vi "Choreo_ChoreoDifferential_LoadTrajectoryString.vi"(11 "trajectoryJsonString":string) -> (0 "Error":bool, 3 "ChoreoTrajectoryDifferential":T1)   [LabVIEW 2019, in "ChoreoLib.lvlib"]
doc: "Parse a Differential choreo trajectory from a JSON formatted string. \n\nInputs: \n - trajectoryJsonString - string- The string containing the choreo trajectory. Note that files may have a .TRAJ extension. These are actually internally formatted as JSON files.\n\nOutputs:\n - ChoreoTrajectorySwerve - cluster - Trajectory read from JSON file.\n - Error - boolean - TRUE if an error occured."
uses:
  ChoreoLib.lvlib
  TypeDef/ChoreoEventMarker.ctl
  TypeDef/ChoreoTrajectoryDifferential.ctl
  TypeDef/ChoreoDifferentialSample.ctl
panel:
  out "nameErr":bool
  out "EventsEmpty":bool
  out "EventMarkers":T3[](array[typedef])
  out "splitsErr":bool
  out "version":i32
  out "sampleType":string
  out "VersionErr":bool
  out "SampleTypeErr":bool
  in  "?":T4(array[cluster])
  out "sampleError":bool
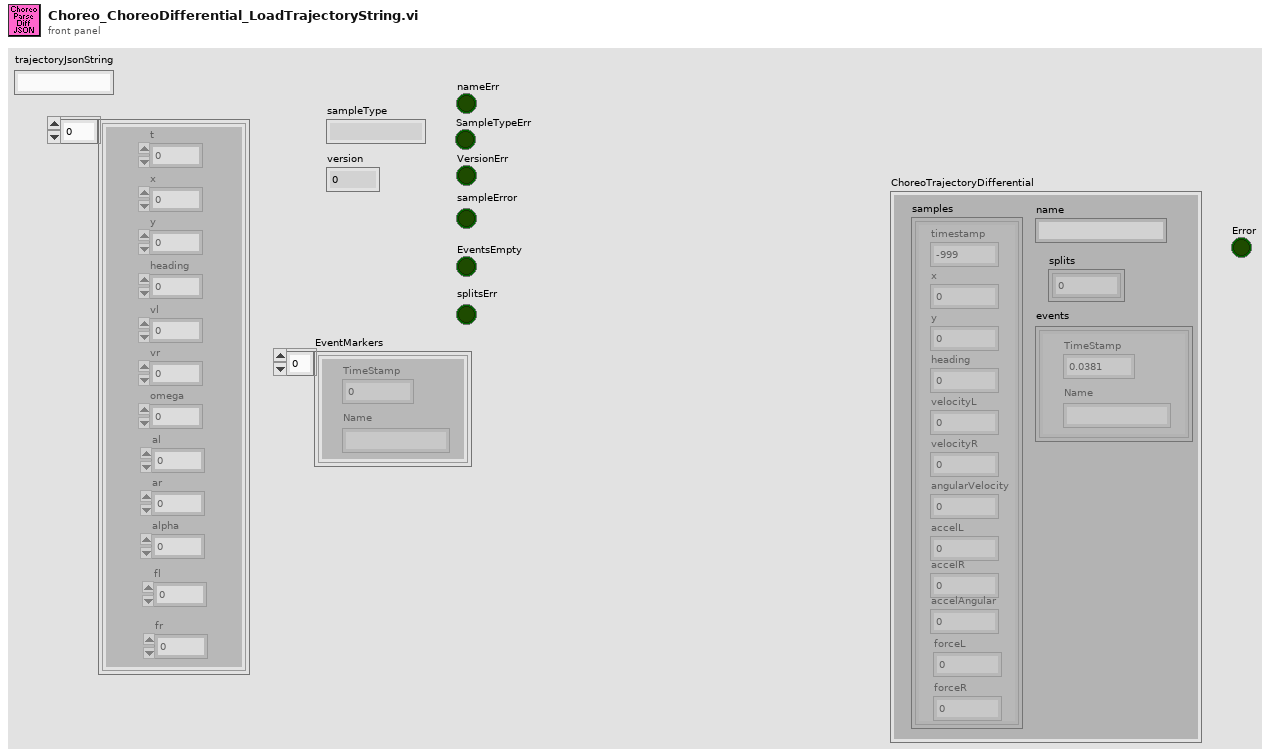
[diagram p1: front panel]
types:
  T1 = typedef "ChoreoLib.lvlib/ChoreoTrajectoryDifferential.ctl" = cluster{"name":string, "samples":T2[], "splits":i32[], "events":T3[]}
  T2 = typedef "ChoreoLib.lvlib/ChoreoDifferentialSample.ctl" = cluster{"timestamp":dbl, "x":dbl, "y":dbl, "heading":dbl, "velocityL":dbl, "velocityR":dbl, "angularVelocity":dbl, "accelL":dbl, "accelR":dbl, "accelAngular":dbl, "forceL":dbl, "forceR":dbl}
  T3 = typedef "ChoreoLib.lvlib/ChoreoEventMarker.ctl" = cluster{"TimeStamp":dbl, "Name":string}
  T4 = cluster{"t":dbl, "x":dbl, "y":dbl, "heading":dbl, "vl":dbl, "vr":dbl, "omega":dbl, "al":dbl, "ar":dbl, "alpha":dbl, "fl":dbl, "fr":dbl}[]
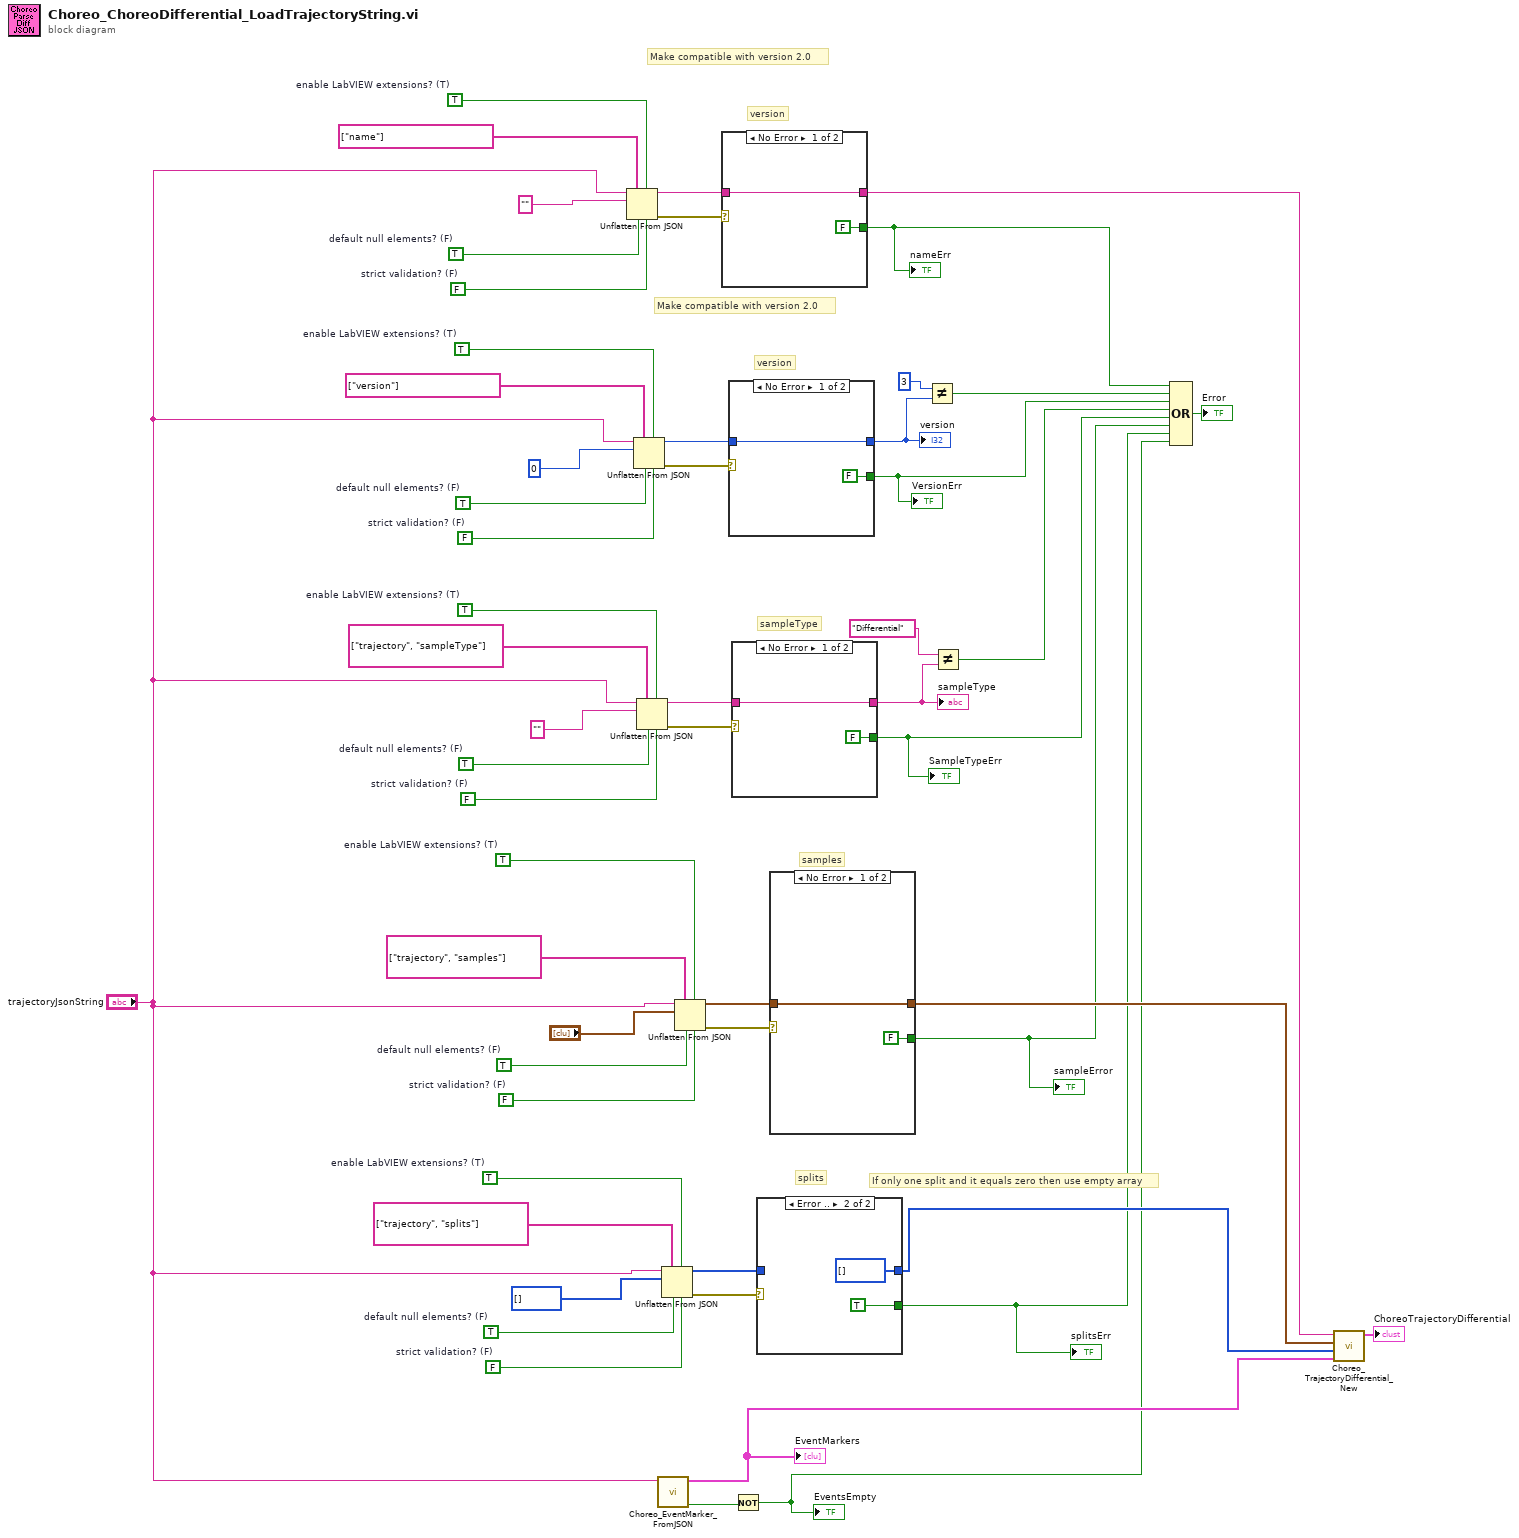
[diagram p0: block diagram]
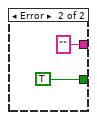
[diagram p2: hidden frame]
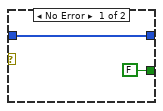
[diagram p3: hidden frame]
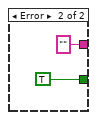
[diagram p4: hidden frame]
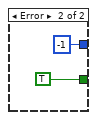
[diagram p5: hidden frame]
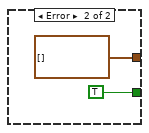
[diagram p6: hidden frame]
diagram:
  w20 = FALSE  # strict validation? (F)
  w21 = TRUE  # default null elements? (F)
  w22 = TRUE  # enable LabVIEW extensions? (T)
  w30 = FALSE  # strict validation? (F)
  w31 = TRUE  # default null elements? (F)
  w32 = TRUE  # enable LabVIEW extensions? (T)
  w37 = FALSE  # strict validation? (F)
  w38 = TRUE  # default null elements? (F)
  w39 = TRUE  # enable LabVIEW extensions? (T)
  w44 = FALSE  # strict validation? (F)
  w45 = TRUE  # default null elements? (F)
  w46 = TRUE  # enable LabVIEW extensions? (T)
  w51 = FALSE  # strict validation? (F)
  w52 = TRUE  # default null elements? (F)
  w53 = TRUE  # enable LabVIEW extensions? (T)
  # "version"
  # "Make compatible with version 2.0"
  # "If only one split and it equals zero then use empty array"
  # "splits"
  # "samples"
  # "sampleType"
  # "version"
  # "Make compatible with version 2.0"
  n1 = Unflatten From JSON(path=string[] ["name"] ("path 7"), enable LabVIEW extensions? (T)=w22, JSON string="trajectoryJsonString", type and defaults="", default null elements? (F)=w21, strict validation? (F)=w20) -> (value=w23:string, error out=w24:errorcluster)  [unwired: 1 in]
  n2 = Unflatten From JSON(path=string[] ["version"] ("path 7"), enable LabVIEW extensions? (T)=w46, JSON string="trajectoryJsonString", type and defaults=0, default null elements? (F)=w45, strict validation? (F)=w44) -> (value=w47:i32, error out=w48:errorcluster)  [unwired: 1 in]
  n3 = Unflatten From JSON(path=string[] ["trajectory", "sampleType"] ("path 7"), enable LabVIEW extensions? (T)=w39, JSON string="trajectoryJsonString", type and defaults="", default null elements? (F)=w38, strict validation? (F)=w37) -> (value=w40:string, error out=w41:errorcluster)  [unwired: 1 in]
  n4 = call "Choreo_EventMarker_FromJSON.vi"("JSON String"="trajectoryJsonString") -> ("Exists"=w27:bool, "EventMarkers"=w5:T3[])  [unwired: 9 in]
  "EventMarkers" <- w5
  n5 = Unflatten From JSON(path=string[] ["trajectory", "splits"] ("path 7"), enable LabVIEW extensions? (T)=w32, JSON string="trajectoryJsonString", type and defaults=i32[] [], default null elements? (F)=w31, strict validation? (F)=w30) -> (value=w33:i32[], error out=w34:errorcluster)  [unwired: 1 in]
  n6 = Unflatten From JSON(path=string[] ["trajectory", "samples"] ("path 7"), enable LabVIEW extensions? (T)=w53, JSON string="trajectoryJsonString", type and defaults="?", default null elements? (F)=w52, strict validation? (F)=w51) -> (value=w54:T4, error out=w55:errorcluster)  [unwired: 1 in]
  n7 = case shown="No Error" w24 {
    tunnel: w23 -> [w56 _]
    tunnel: [FALSE TRUE] -> w15
    tunnel: [w56 ""] -> w16
    frame No Error {
    }
    frame Error {
    }
  }
  "nameErr" <- w15
  n8 = case shown="No Error" w48 {
    tunnel: w47 -> [w60 _]
    tunnel: [FALSE TRUE] -> w11
    tunnel: [w60 -1] -> w14
    frame No Error {
    }
    frame Error {
    }
  }
  "VersionErr" <- w11
  "version" <- w14
  n9 = case shown="No Error" w41 {
    tunnel: w40 -> [w64 _]
    tunnel: [FALSE TRUE] -> w7
    tunnel: [w64 ""] -> w10
    frame No Error {
    }
    frame Error {
    }
  }
  "SampleTypeErr" <- w7
  "sampleType" <- w10
  n10 = Not(x=w27) -> (.not. x?=w3:bool)
  "EventsEmpty" <- w3
  n11 = case shown="Error .." w34 {
    tunnel: w33 -> [w68 _]
    tunnel: [FALSE TRUE] -> w4
    tunnel: [w68 i32[] []] -> w25
    frame No Error {
    }
    frame Error {
    }
  }
  "splitsErr" <- w4
  n12 = case shown="No Error" w55 {
    tunnel: w54 -> [w72 _]
    tunnel: [FALSE TRUE] -> w6
    tunnel: [w72 T2[] []] -> w26
    frame No Error {
    }
    frame Error {
    }
  }
  "sampleError" <- w6
  n13 = Not Equal?(x=3, y=w14) -> (x != y?=w12:bool)
  n14 = Not Equal?(x="Differential", y=w10) -> (x != y?=w8:bool)
  n15 = Compound Arithmetic op=OR(w15, w12, w11, w8, w7, w6, w4, w3) -> (→"Error":bool)
  n16 = call "Choreo_TrajectoryDifferential_New.vi"("events"=w5, "splits"=w25, "samples"=w26, "name"=w16) -> ("ChoreoTrajectoryDifferential"=→"ChoreoTrajectoryDifferential":T1)  [unwired: 7 in]
